vi "Differential_delay_line_configuration_Mezzaninev56_initialize_Sockets.vi"(0 "connection ID":refnum<k5>, 3 "error in (no error)":errorcluster) -> (6 "connection ID out":refnum<k5>, 9 "error out 2":errorcluster)   [LabVIEW 2012]
panel:
  out "data out serial":string
  out "hex integer string":string
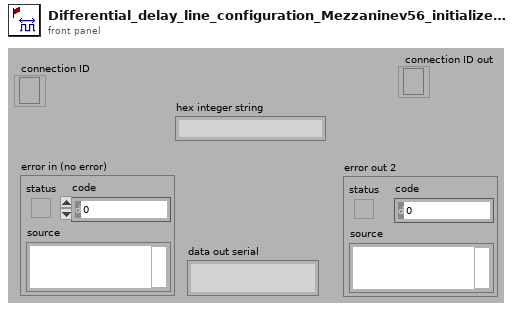
[diagram p1: front panel]
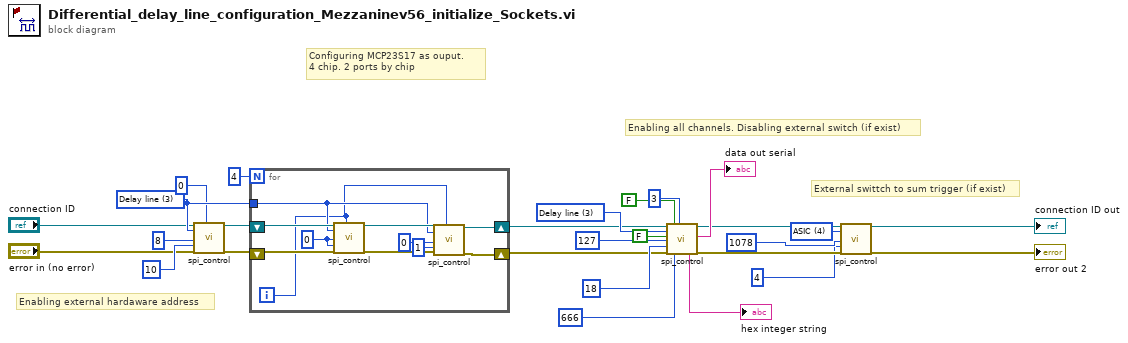
[diagram p0: block diagram]
diagram:
  w6 = u16 4 items=["Attenuation", "Clipping", "Enable channel", "Delay line", "ASIC"] ("Device")
  w24 = u16 3 items=["Attenuation", "Clipping", "Enable channel", "Delay line", "ASIC"] ("Device")
  w16 = u16 3 items=["Attenuation", "Clipping", "Enable channel", "Delay line", "ASIC"] ("Device")
  # "External swittch to sum trigger (if exist)"
  # "Enabling external hardaware address"
  # "Configuring MCP23S17 as ouput.\n4 chip. 2 ports by chip"
  # "Enabling all channels. Disabling external switch (if exist)"
  n1 = call "spi_control.vi"("connection ID"="connection ID", "Device"=w16, "Data"=8, "Register or channel"=10, "error in"="error in (no error)", "chip delay"=0) -> ("connection ID out"=w15:refnum<k5>, "error out 2"=w14:errorcluster)  [unwired: 6 in, 6 out]
  n2 = for {
    N: 4 -> [_]
    tunnel: w16 -> [w32]
    shift-right: [w38] -> w21
    shift-left: w14 -> [w36]
    shift-right: [w33] -> w20
    shift-left: w15 -> [w35]
    i -> [w28]
    w30 = 0 ("Data")
    n3 = call "spi_control.vi"("connection ID"=w35, "Device"=w32, "Data"=w30, "Register or channel"=w30, "error in"=w36, "chip delay"=w28) -> ("connection ID out"=w34:refnum<k5>, "error out 2"=w37:errorcluster)  [unwired: 6 in, 6 out]
    n4 = call "spi_control.vi"("connection ID"=w34, "Device"=w32, "Data"=0, "Register or channel"=1, "error in"=w37, "chip delay"=w28) -> ("connection ID out"=w33:refnum<k5>, "error out 2"=w38:errorcluster)  [unwired: 6 in, 6 out]
  }
  n5 = call "spi_control.vi"("connection ID"=w20, "Device"=w24, "Read/#write"=FALSE, "Data"=127, "Register or channel"=18, "error in"=w21, "Read physical"=FALSE, "Id in"=666, "chip delay"=3 ("Channel delay")) -> ("hex integer string"=→"hex integer string":string, "connection ID out"=w7:refnum<k5>, "data out serial"=→"data out serial":string, "error out 2"=w8:errorcluster)  [unwired: 3 in, 4 out]
  n6 = call "spi_control.vi"("connection ID"=w7, "Device"=w6, "Data"=1078, "Register or channel"=4, "error in"=w8) -> ("connection ID out"=→"connection ID out":refnum<k5>, "error out 2"=→"error out 2":errorcluster)  [unwired: 7 in, 6 out]
